vi "Create.vi"(10 "Logger Status":T1) -> (3 "Logger Status Value out":refnum<class "Logger Status Value.lvclass">)   [LabVIEW 2020, in "VolatusHistorian.lvlib" / "Logger Status Value.lvclass"]
uses:
  Logger Status Value.lvclass
  Logger Status Value.lvclass/Logger Status Value.ctl
  Logger Status.ctl
  VolatusHistorian.lvlib
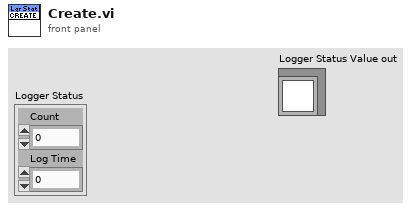
[diagram p1: front panel]
types:
  T1 = typedef "VolatusHistorian.lvlib/Logger Status.ctl" = cluster{"Count":i32, "Log Time":dbl}
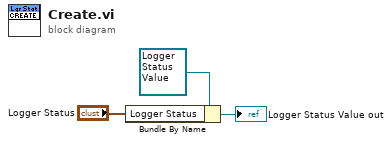
[diagram p0: block diagram]
diagram:
  n1 = Bundle By Name(cluster=refnum<class "Logger Status Value.lvclass"> refnum ("Logger Status Value in"), "Logger Status"="Logger Status") -> (→"Logger Status Value out":refnum<class "Logger Status Value.lvclass">)
